vi "Custom TCP Connection Handler.vi"(4 "TCP Network Connection in":refnum<k5>, 5 "Debugging":bool, 7 "Error In":errorcluster) -> (3 "Error Out":errorcluster)   [LabVIEW 2020, in "Startup Processes.lvlib"]
uses:
  Startup Processes.lvlib
  toolbox/Standard Signalling/ude_Stop Application/ude_Stop Application.lvlib
  toolbox/Standard Signalling/ude_Handle Errors/ude_Handle Errors.lvlib
  toolbox/Error Correction/Error Correction.lvlib
  _typedefs/Custom TCP Handler States.ctl
  _typedefs/Custom Remote Access Error Codes.ctl
  _classes/Remote Access Commands/Remote Access Commands.lvclass
  _typedefs/JSON Response Cluster.ctl
panel:
  out "Response out":T1
  out "JSON Command String":string
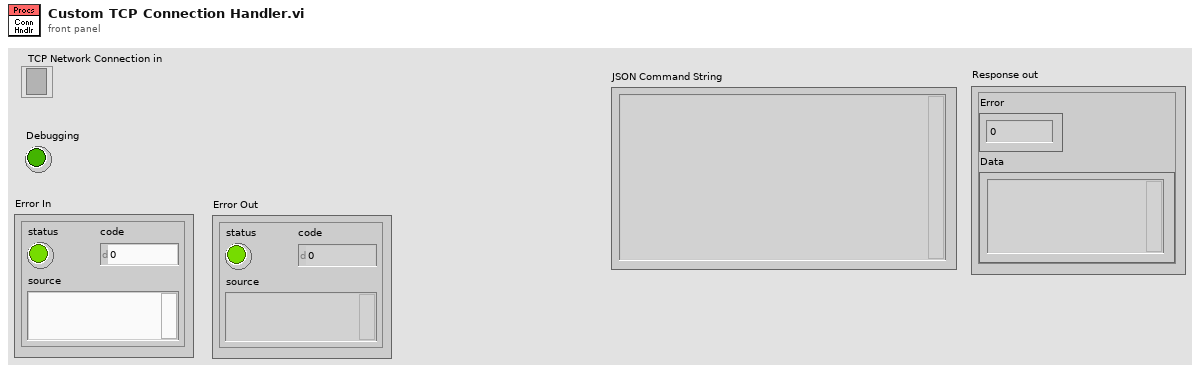
[diagram p1: front panel]
types:
  T1 = typedef "Startup Processes.lvlib/JSON Response Cluster.ctl" = cluster{"Error":i32, "Data":string}
  T2 = typedef "Startup Processes.lvlib/Custom TCP Handler States.ctl" = enum16{"Read Data Packet", "Process Command", "Send Response", "Stop Handler"}
  T3 = enum32{"Invalid", "Standard", "Closed", "Hidden", "Minimized", "Maximized"}
  T4 = typedef "Startup Processes.lvlib/Custom Remote Access Error Codes.ctl" = enum16{"No Error", "CRC Error", "Update Failed"}
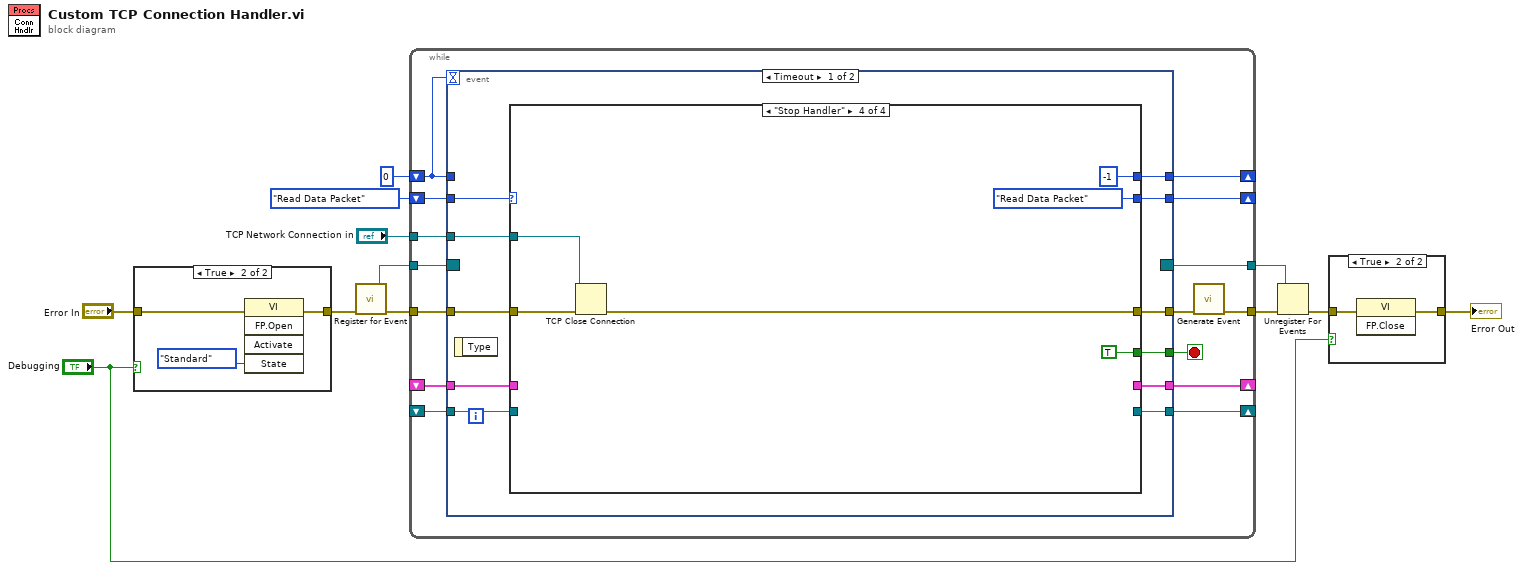
[diagram p0: block diagram]
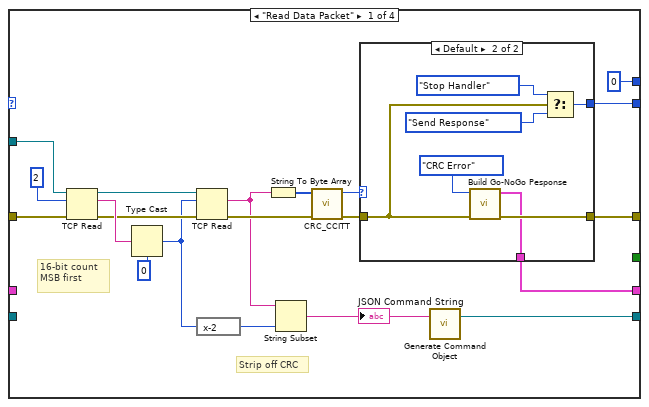
[diagram p3: hidden frame]
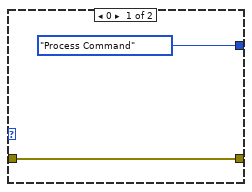
[diagram p4: hidden frame]
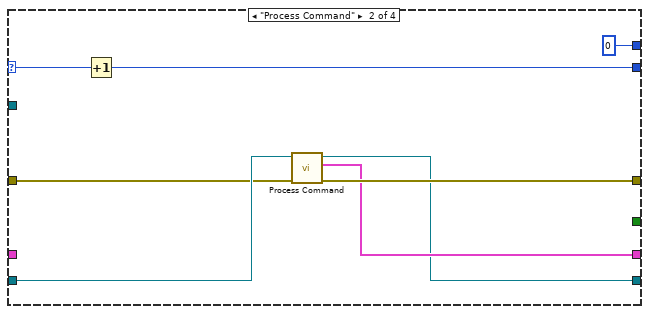
[diagram p5: hidden frame]
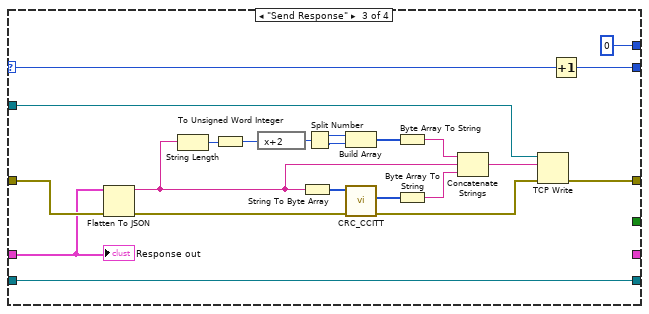
[diagram p6: hidden frame]
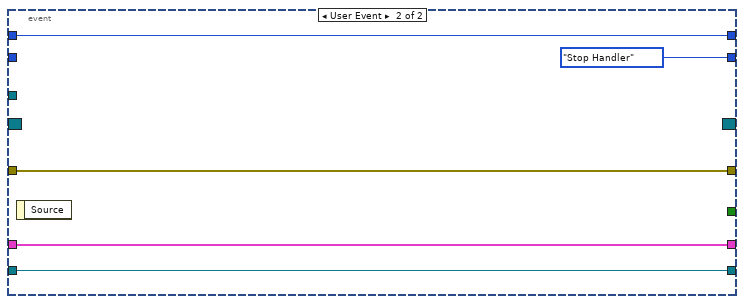
[diagram p7: hidden frame]
diagram:
  n1 = case shown="True" "Debugging" {
    tunnel: "Error In" -> [w13 w16]
    tunnel: [w13 w15] -> w2
    frame False {
    }
    frame True {
      n2 = invoke class="VI" method="FP.Open"(error in=w16, "State"=T3."Standard") -> (error out=w15:errorcluster)  [unwired: 3 in, 4 out]
    }
  }
  n3 = call "Register for Event.vi"("Error In"=w2) -> ("Error Out"=w9:errorcluster, "sys"=w10:refnum<event-registration>)  [unwired: 5 in]
  n4 = while {
    tunnel: "TCP Network Connection in" -> [w31]
    tunnel: w10 -> [w29]
    tunnel: [w28] -> w12
    shift-right: [w26] -> _
    shift-left: 0 -> [w25]
    shift-right: [w21] -> _
    shift-left: Custom_TCP_Handler_States."Read Data Packet" -> [w24]
    shift-right: [w20] -> _
    shift-left: _ -> [w19]
    shift-right: [w17] -> _
    shift-left: _ -> [w18]
    tunnel: w9 -> [w27]
    tunnel: [w23] -> w11
    stop <- w30 stop-if-true
    n5 = event shown="[0] Timeout" {
      selector: w29 -> [_ _]
      dyn-events: [_ _] -> w28
      timeout: w25 -> [_ _]
      tunnel: w31 -> [w41 _]
      tunnel: [w33 _] -> w30
      tunnel: w27 -> [w40 w108]
      tunnel: [w39 w108] -> w22
      tunnel: [w38 w112] -> w26
      tunnel: w25 -> [_ w112]
      tunnel: w24 -> [w42 _]
      tunnel: [w37 Custom_TCP_Handler_States."Stop Handler"] -> w21
      tunnel: [w32 w111] -> w20
      tunnel: w19 -> [w36 w111]
      tunnel: w18 -> [w35 w110]
      tunnel: [w34 w110] -> w17
      event Timeout {
        n6 = event-data() -> ()  [unwired: 1 in, 1 out]
        n7 = case shown="\"Stop Handler\"" w42 {
          selector: w42 -> [_ w78 w80 _]
          tunnel: w41 -> [w62 _ w86 w105]
          tunnel: w40 -> [w61 w75 w99 w104]
          tunnel: [w45 w74 w83 w103] -> w39
          tunnel: [0 0 0 -1] -> w38
          tunnel: [w51 w77 w100 Custom_TCP_Handler_States."Read Data Packet"] -> w37
          tunnel: w36 -> [_ w76 w81 _]
          tunnel: w35 -> [_ _ w98 _]
          tunnel: [w50 w73 _ _] -> w34
          tunnel: [_ _ _ TRUE] -> w33
          tunnel: [w44 w72 w81 _] -> w32
          frame "Read Data Packet" {
            # "Strip off CRC"
            # "16-bit count MSB first"
            n8 = TCP Read(connection ID=w62, bytes to read=2, error in (no error)=w61) -> (connection ID out=w57:refnum<k5>, data out=w58:string, error out=w56:errorcluster)  [unwired: 2 in]
            n9 = Type Cast(type=u16 0, x=w58) -> (*(type *) &x=w48:u16)
            n10 = TCP Read(connection ID=w57, bytes to read=w48, error in (no error)=w56) -> (data out=w49:string, error out=w55:errorcluster)  [unwired: 2 in, 1 out]
            n11 = expression code="x-2"(w48) -> (w47:u16)
            n12 = String To Byte Array(string=w49) -> (unsigned byte array=w54:u8[])
            n13 = String Subset(string=w49, length (rest)=w47) -> (substring=w43:string)  [unwired: 1 in]
            "JSON Command String" <- w43
            n14 = call "CRC_CCITT.vi"("error in (no error)"=w55, "unsigned byte array"=w54) -> ("error out"=w46:errorcluster, "CRC-CCITT"=w53:u16)  [unwired: 3 in, 1 out]
            n15 = case shown="Default" w53 {
              tunnel: [Custom_TCP_Handler_States."Process Command" w68] -> w51
              tunnel: [_ w69] -> w50
              tunnel: w46 -> [w63 w66]
              tunnel: [w63 w70] -> w45
              frame 0 {
              }
              frame Default {
                n16 = call "Build Go-NoGo Pesponse.vi"("error in (no error)"=w66, "Error"=Custom_Remote_Access_Error_Codes."CRC Error") -> ("error out"=w70:errorcluster, "Response"=w69:T1)  [unwired: 4 in]
                n17 = Select(t=Custom_TCP_Handler_States."Stop Handler", s=w66, f=Custom_TCP_Handler_States."Send Response") -> (s? t:f=w68:T2)
              }
            }
            n18 = call "Generate Command Object.vi"("data in"=w43) -> ("Remote Access Commands.lvclass"=w44:refnum<class "Remote Access Commands.lvclass">)  [unwired: 2 in]
          }
          frame "Process Command" {
            n19 = Increment(x=w78) -> (x+1=w77:T2)
            n20 = call-dynamic "Process Command.vi"("error in (no error)"=w75, "Remote Access Commands in"=w76) -> ("error out"=w74:errorcluster, "Response out"=w73:T1, "Remote Access Commands out"=w72:refnum<class "Remote Access Commands.lvclass">)  [unwired: 3 in]
          }
          frame "Send Response" {
            n21 = Flatten To JSON(anything=w98, error in (no error)=w99) -> (JSON string=w82:string, 11:w94:errorcluster)  [unwired: 1 in]
            n22 = String Length(string=w82) -> (length=w93:i32)
            n23 = To Unsigned Word Integer(number=w93) -> (unsigned 16bit integer=w92:u16)
            n24 = expression code="x+2"(w92) -> (w91:u16)
            n25 = String To Byte Array(string=w82) -> (unsigned byte array=w97:u8[])
            n26 = Split Number(x=w91) -> (hi(x)=w90:u8, lo(x)=w89:u8)
            n27 = Build Array(w90, w89) -> (w88:u8[])
            n28 = call "CRC_CCITT.vi"("error in (no error)"=w94, "unsigned byte array"=w97) -> ("error out"=w84:errorcluster, "CRC array"=w96:u8[])  [unwired: 3 in, 1 out]
            n29 = Byte Array To String(unsigned byte array=w88) -> (string=w87:string)
            n30 = Byte Array To String(unsigned byte array=w96) -> (string=w95:string)
            n31 = Concatenate Strings(w87, w82, w95) -> (w85:string)
            n32 = TCP Write(connection ID=w86, data in=w85, error in (no error)=w84) -> (error out=w83:errorcluster)  [unwired: 1 in, 2 out]
            n33 = Increment(x=w80) -> (x+1=w100:T2)
            "Response out" <- w98
          }
          frame "Stop Handler" {
            n34 = TCP Close Connection(connection ID=w105, error in (no error)=w104) -> (error out=w103:errorcluster)  [unwired: 1 in, 1 out]
          }
        }
      }
      event User Event {
        n35 = event-data() -> ()  [unwired: 1 in, 1 out]
      }
    }
    n36 = call "Generate Event.vi"("Error In"=w22) -> ("Error Out"=w23:errorcluster)  [unwired: 6 in]
  }
  n37 = Unregister For Events(event registration refnum=w12, error in=w11) -> (error out=w6:errorcluster)
  n38 = case shown="True" "Debugging" {
    tunnel: w6 -> [w113 w115]
    tunnel: [w113 w114] -> w4
    frame False {
    }
    frame True {
      n39 = invoke class="VI" method="FP.Close"(error in=w115) -> (error out=w114:errorcluster)  [unwired: 2 in, 2 out]
    }
  }
  "Error Out" <- w4
